vi "Find User Rating.vi"(10 "Names":T1[](array[typedef]), 11 "String":string) -> (1 "Found?":bool, 3 "Score":dbl)   [LabVIEW 2014]
uses:
  User Score Update.ctl
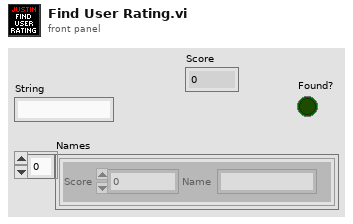
[diagram p1: front panel]
types:
  T1 = typedef "User Score Update.ctl" = cluster{"Score":dbl, "Name":string}
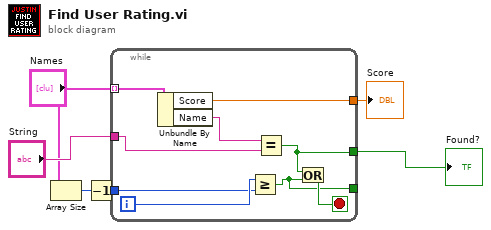
[diagram p0: block diagram]
diagram:
  n1 = Array Size(array="Names") -> (size(s)=w3:i32)
  n2 = Decrement(x=w3) -> (x-1=w2:i32)
  n3 = while {
    tunnel: "Names" -> [w14] mode=indexing
    tunnel: "String" -> [w15]
    tunnel: [w12] -> w5
    tunnel: w2 -> [w10]
    tunnel: [w8] -> _
    tunnel: [w7] -> w1
    i -> [w11]
    stop <- w9 stop-if-true
    n4 = Unbundle By Name(w14) -> ("Score"=w12:dbl, "Name"=w13:string)
    n5 = Greater Or Equal?(x=w11, y=w10) -> (x >= y?=w8:bool)
    n6 = Equal?(x=w13, y=w15) -> (x = y?=w7:bool)
    n7 = Or(x=w7, y=w8) -> (x .or. y?=w9:bool)
  }
  "Score" <- w5
  "Found?" <- w1
